vi "SECoP_dataGetInteger.vi"(7 "Position":u32, 8 "error in (no error)":errorcluster, 9 "Index":u32, 10 "SECoP_dataPtr":T1 {"ptr64" format="%.0x"; "ptr32" format="%.0x"}, 11 "DLL path (in)":T2) -> (0 "error out":errorcluster, 2 "Value":i64, 3 "DLL path (out)":T2)   [LabVIEW 2023, in "SECoP.lvlib"]
doc: "Call <b>\"SECoP_dataGetInteger.vi\"</b> to access the numeric value (integer or scaled of SECoP_dataPtr).\n\n<b>DLL path</b> input and output of cluster from \"SECoP-Initialize.vi\"\n<b>SECoP_dataPtr</b> data to access\n<b>Position</b> points to a virtual flattened entry of the data type\n<b>Index</b> zero based index into array type or 0 for single numeric type\n<b>Value</b> numeric integer or unscaled value"
uses:
  SECoP.lvlib
  SECoP-libraries.ctl
  SECoP-data.ctl
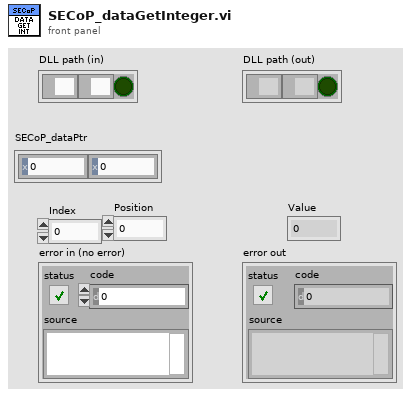
[diagram p1: front panel]
types:
  T1 = typedef "SECoP.lvlib/SECoP-data.ctl" = cluster{"ptr32":u32, "ptr64":u64}
  T2 = typedef "SECoP.lvlib/SECoP-libraries.ctl" = cluster{"serverDLL":path, "variantDLL":path, "cleanup_mode":bool}
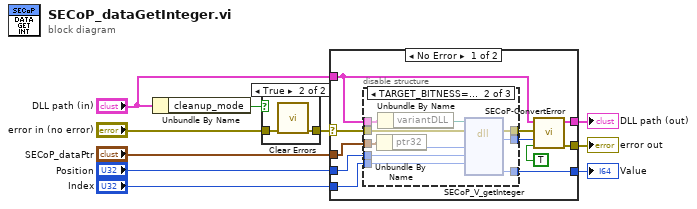
[diagram p0: block diagram]
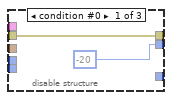
[diagram p3: hidden frame]
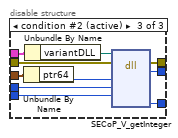
[diagram p4: hidden frame]
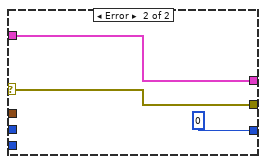
[diagram p5: hidden frame]
diagram:
  n1 = Unbundle By Name("DLL path (in)") -> ("cleanup_mode"=w7:bool)
  n2 = case shown="True" w7 {
    tunnel: "error in (no error)" -> [w11 w13]
    tunnel: [w11 w12] -> w5
    frame False {
    }
    frame True {
      n3 = call <vilib>:"Clear Errors.vi"("error in (no error)"=w13) -> ("error out"=w12:errorcluster)  [unwired: 5 in, 1 out]
    }
  }
  n4 = case shown="No Error" w5 {
    selector: w5 -> [w22 w48]
    tunnel: "DLL path (in)" -> [w14 w49]
    tunnel: [w23 w49] -> w9
    tunnel: [w24 w48] -> w8
    tunnel: "Position" -> [w18 _]
    tunnel: "Index" -> [w17 _]
    tunnel: [w16 i64 0 ("Value")] -> w2
    tunnel: "SECoP_dataPtr" -> [w15 _]
    frame No Error {
      n5 = disable-structure shown="TARGET_BITNESS==32" {
        disable-tunnel: w22 -> [w25 w36 w46]
        disable-tunnel: w14 -> [_ w35 w45]
        disable-tunnel: [w25 w34 w44] -> w21
        disable-tunnel: [-20 w33 w43] -> w20
        disable-tunnel: w18 -> [_ w32 w42]
        disable-tunnel: w17 -> [_ w31 w41]
        disable-tunnel: [_ w30 w40] -> w16
        disable-tunnel: w15 -> [_ w28 w38]
        frame condition #0 {
        }
        frame condition #1 {
          n6 = Unbundle By Name(w28) -> ("ptr32"=w29:u32)
          n7 = Unbundle By Name(w35) -> ("variantDLL"=w27:path)
          n8 = dll-call lib="Z:/Praktische_Aufgaben/SECoP-LabVIEW2015/32bit/SECoP32.dll" fn="SECoP_V_getInteger"(path in=w27, error in=w36, "Data"=w29, "Position"=w32, "Index"=w31) -> (error out=w34:errorcluster, "return type"=w33:i32, "Value"=w30:i64)  [unwired: 5 in, 1 out]
        }
        frame condition #2 (active) {
          n9 = Unbundle By Name(w38) -> ("ptr64"=w39:u64)
          n10 = Unbundle By Name(w45) -> ("variantDLL"=w37:path)
          n11 = dll-call lib="Z:/Praktische_Aufgaben/SECoP-LabVIEW2015/32bit/SECoP32.dll" fn="SECoP_V_getInteger"(path in=w37, error in=w46, "Data"=w39, "Position"=w42, "Index"=w41) -> (error out=w44:errorcluster, "return type"=w43:i32, "Value"=w40:i64)  [unwired: 5 in, 1 out]
        }
      }
      n12 = call "SECoP-ConvertError.vi"("return is boolean"=TRUE, "return code"=w20, "error in (no error)"=w21, "DLL path (in)"=w14) -> ("error out"=w24:errorcluster, "DLL path (out)"=w23:T2)  [unwired: 6 in]
    }
    frame Error {
    }
  }
  "DLL path (out)" <- w9
  "error out" <- w8
  "Value" <- w2
